vi "Destroy InverterLUT Dict Ref.vi"(8 "error in (no error)":errorcluster, 11 "Main in":refnum<class "Main.lvclass">) -> (0 "error out":errorcluster, 3 "Main out":refnum<class "Main.lvclass">)   [LabVIEW 2019, in "Main.lvclass"]
doc: "Developed by Kevin Thompson\nkevin@thompsonengineering.net\n\nCopyright 2020\nThompson Engineering, LLC"
uses:
  Main.lvclass
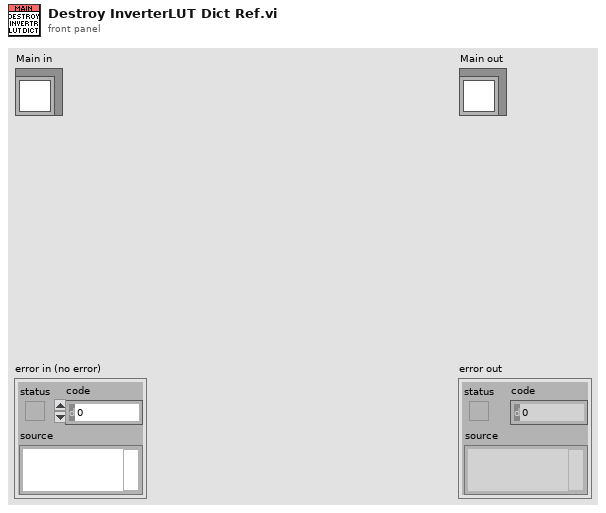
[diagram p1: front panel]
types:
  T1 = typedef "TD Dynamic CVT DVR--ref.ctl" = refnum<data-value>
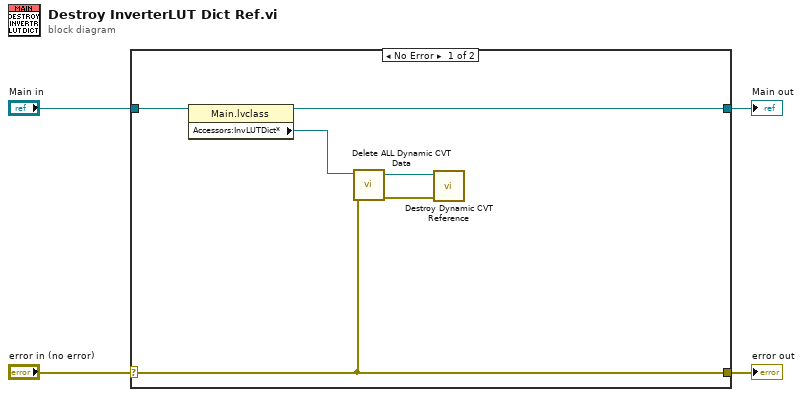
[diagram p0: block diagram]
diagram:
  n1 = case shown="No Error" "error in (no error)" {
    selector: "error in (no error)" -> [w5 w12]
    tunnel: [w5 w12] -> w3
    tunnel: [w9 w11] -> w1
    tunnel: "Main in" -> [w10 w11]
    frame No Error {
      n2 = property class="Main.lvclass"(reference=w10) -> (reference out=w9:refnum<class "Main.lvclass">, "Accessors:InvLUTDict*"=w8:T1)  [unwired: 1 in, 1 out]
      n3 = call <vilib>:"Delete ALL Dynamic CVT Data.vi"("error in (no error)"=w5, "dCVT DVR"=w8) -> ("error out"=w6:errorcluster, "dCVT DVR out"=w7:T1)  [unwired: 8 in]
      n4 = call <vilib>:"Destroy Dynamic CVT Reference.vi"("error in (no error)"=w6, "dCVT DVR"=w7) -> ()  [unwired: 8 in, 2 out]
    }
    frame Error {
    }
  }
  "error out" <- w3
  "Main out" <- w1
